vi "test_MSS multiple start stop mismatch1.vi"(8 "Error In":errorcluster) -> (0 "Error Out":errorcluster)   [LabVIEW 2023]
uses:
  Measure and Stimulus Subsystems.lvclass
panel:
  out "Powersensor Chart":waveform(dbl)(graph)
  in  "Stop":bool
  out "Photosensor Chart":waveform(dbl)(graph)
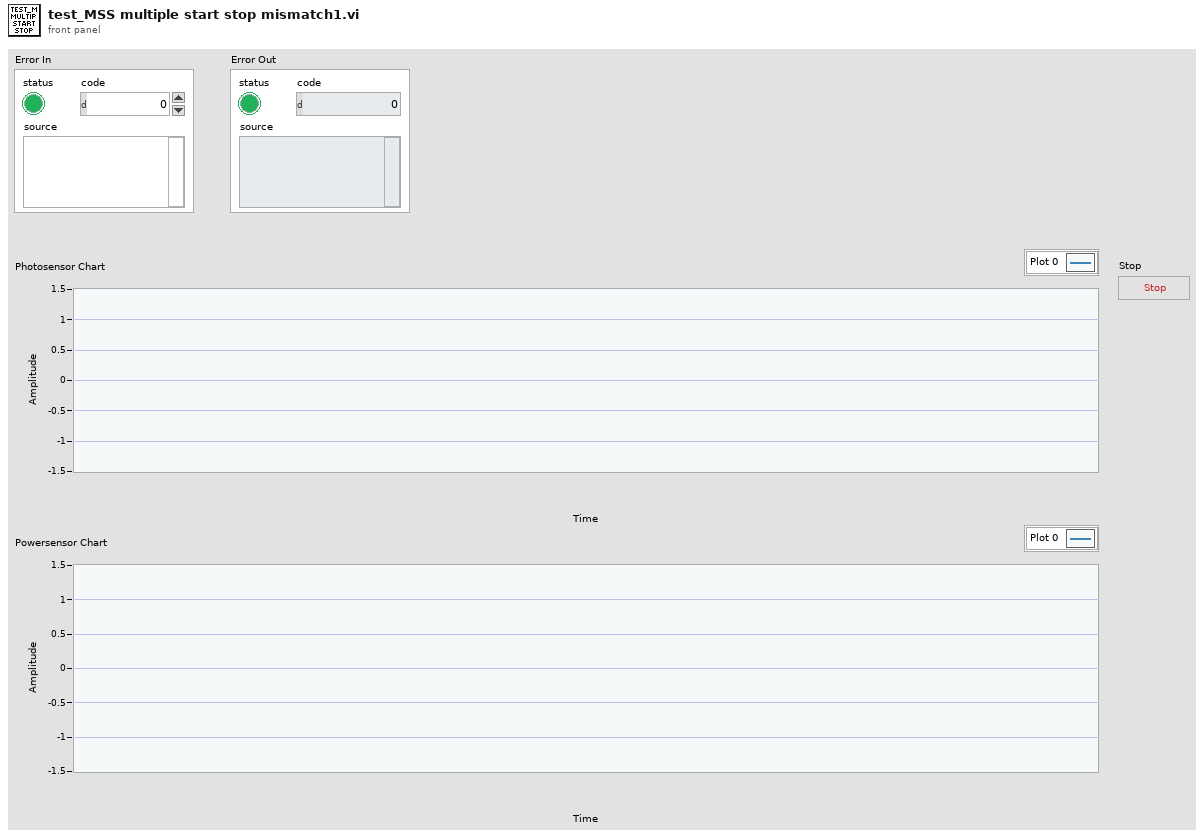
[diagram p1: front panel]
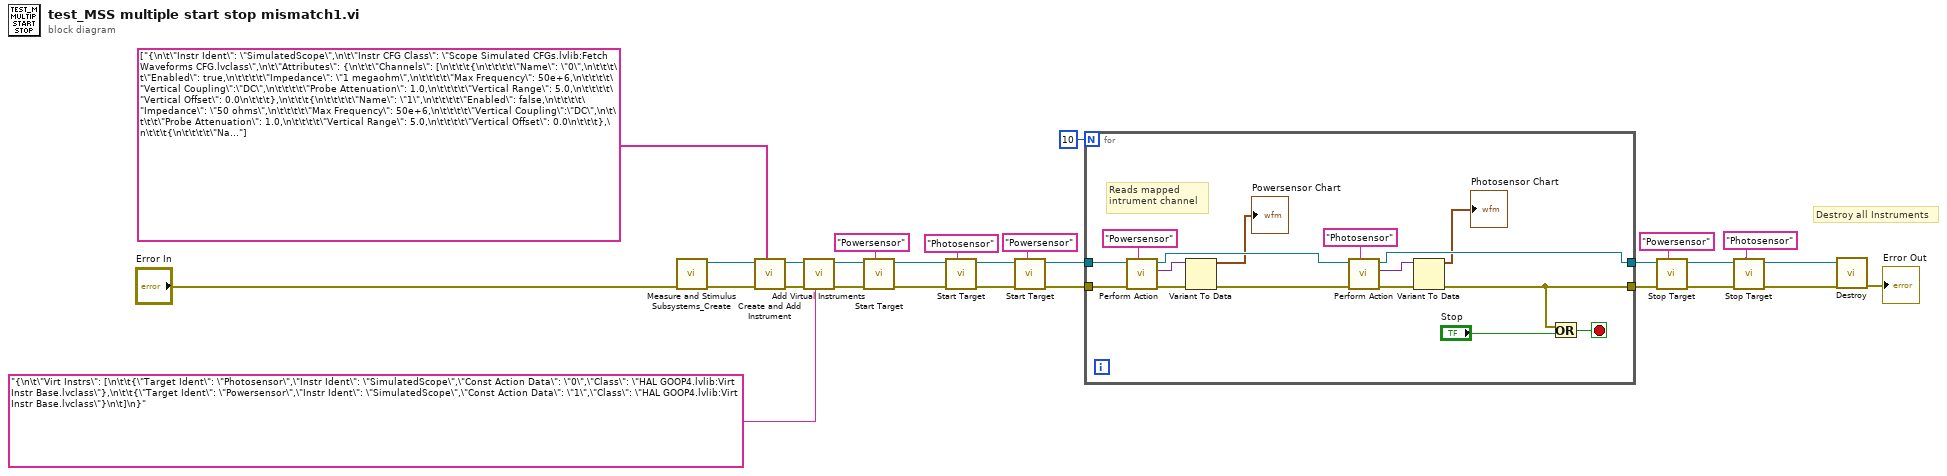
[diagram p0: block diagram]
diagram:
  # "Destroy all Instruments"
  n1 = call "Measure and Stimulus Subsystems_Create.vi"("Error In"="Error In") -> ("Error Out"=w27:errorcluster, "reference out"=w28:refnum<class "Measure and Stimulus Subsystems.lvclass">)  [unwired: 9 in]
  n2 = call "Create and Add Instrument.vi"("Physical Intr Configs"=string[] ["{\n\t\"Instr Ident\": \"SimulatedScope\",\n\t\"Instr CFG Class\": \"Scope Simulated CFGs.lvlib:Fetch Waveforms CFG.lvclass\",\n\t\"Attributes\": {\n\t\t\"Channels\": [\n\t\t\t{\n\t\t\t\t\"Name\": \"0\",\n\t\t\t\t\"Enabled\": true,\n\t\t\t\t\"Impedance\": \"1 megaohm\",\n\t\t\t\t\"Max Frequency\": 50e+6,\n\t\t\t\t\"Vertical Coupling\":\"DC\",\n\t\t\t\t\"Probe Attenuation\": 1.0,\n\t\t\t\t\"Vertical Range\": 5.0,\n\t\t\t\t\"Vertical Offset\": 0.0\n\t\t\t},\n\t\t\t{\n\t\t\t\t\"Name\": \"1\",\n\t\t\t\t\"Enabled\": false,\n\t\t\t\t\"Impedance\": \"50 ohms\",\n\t\t\t\t\"Max Frequency\": 50e+6,\n\t\t\t\t\"Vertical Coupling\":\"DC\",\n\t\t\t\t\"Probe Attenuation\": 1.0,\n\t\t\t\t\"Vertical Range\": 5.0,\n\t\t\t\t\"Vertical Offset\": 0.0\n\t\t\t},\n\t\t\t{\n\t\t\t\t\"Name\": \"2\",\n\t\t\t\t\"Enabled\": false,\n\t\t\t\t\"Impedance\": \"50 ohms\",\n\t\t\t\t\"Max Frequency\": 50e+6,\n\t\t\t\t\"Vertical Coupling\":\"DC\",\n\t\t\t\t\"Probe Attenuation\": 1.0,\n\t\t\t\t\"Vertical Range\": 5.0,\n\t\t\t\t\"Vertical Offset\": 0.0\n\t\t\t},\n\t\t\t{\n\t\t\t\t\"Name\": \"3\",\n\t\t\t\t\"Enabled\": true,\n\t\t\t\t\"Impedance\": \"50 ohms\",\n\t\t\t\t\"Max Frequency\": 50e+6,\n\t\t\t\t\"Vertical Coupling\":\"DC\",\n\t\t\t\t\"Probe Attenuation\": 1.0,\n\t\t\t\t\"Vertical Range\": 1.4,\n\t\t\t\t\"Vertical Offset\": 0.0\n\t\t\t},\n\t\t\t{\n\t\t\t\t\"Name\": \"4\",\n\t\t\t\t\"Enabled\": false,\n\t\t\t\t\"Impedance\": \"50 ohms\",\n\t\t\t\t\"Max Frequency\": 50e+6,\n\t\t\t\t\"Vertical Coupling\":\"DC\",\n\t\t\t\t\"Probe Attenuation\": 1.0,\n\t\t\t\t\"Vertical Range\": 5.0,\n\t\t\t\t\"Vertical Offset\": 0.0\n\t\t\t},\n\t\t\t{\n\t\t\t\t\"Name\": \"5\",\n\t\t\t\t\"Enabled\": false,\n\t\t\t\t\"Impedance\": \"50 ohms\",\n\t\t\t\t\"Max Frequency\": 50e+6,\n\t\t\t\t\"Vertical Coupling\":\"DC\",\n\t\t\t\t\"Probe Attenuation\": 1.0,\n\t\t\t\t\"Vertical Range\": 5.0,\n\t\t\t\t\"Vertical Offset\": 0.0\n\t\t\t},\n\t\t\t{\n\t\t\t\t\"Name\": \"6\",\n\t\t\t\t\"Enabled\": false,\n\t\t\t\t\"Impedance\": \"50 ohms\",\n\t\t\t\t\"Max Frequency\": 50e+6,\n\t\t\t\t\"Vertical Coupling\":\"DC\",\n\t\t\t\t\"Probe Attenuation\": 1.0,\n\t\t\t\t\"Vertical Range\": 5.0,\n\t\t\t\t\"Vertical Offset\": 0.0\n\t\t\t},\n\t\t\t{\n\t\t\t\t\"Name\": \"7\",\n\t\t\t\t\"Enabled\": false,\n\t\t\t\t\"Impedance\": \"50 ohms\",\n\t\t\t\t\"Max Frequency\": 50e+6,\n\t\t\t\t\"Vertical Coupling\":\"DC\",\n\t\t\t\t\"Probe Attenuation\": 1.0,\n\t\t\t\t\"Vertical Range\": 5.0,\n\t\t\t\t\"Vertical Offset\": 0.0\n\t\t\t}\n\t\t],\n\t\t\"Horizontal\": {\n\t\t\t\"Enforce Realtime\": true,\n\t\t\t\"Number of Records\": 1,\n\t\t\t\"Min Sample Rate\": 1e+5,\n\t\t\t\"Reference Position\":50, //percent\n\t\t\t\"Min Record Length\":1e+3\n\t\t},\n\t\t\"Acquire\": {\n\t\t\t\"Type\": \"Normal\",\n\t\t\t\"NumSamples\": 1e+3,\n\t\t\t\"Fetch Relative To\": \"Read Pointer\"\n\t\t},\n\t\t\"Export Signal\": {\n\t\t\t\"Signal Identifier\": \"None\",\n\t\t\t\"Signal\": \"None\",\n\t\t\t\"Output Terminal\": \"None\"\n\t\t},\n\t\t\"Trigger\": {\n\t\t\t\"Type\": \"Immediate\",\n\t\t\t\"Slope\": \"Positive\",\n\t\t\t\"Source\": \"RTSI 0\",\n\t\t\t\"Holdoff\": 0.0,\n\t\t\t\"Delay\": 0.0\n\t\t}\n\t}\n}"], "Error In"=w27, "reference in"=w28) -> ("Error Out"=w23:errorcluster, "reference out"=w9:refnum<class "Measure and Stimulus Subsystems.lvclass">)  [unwired: 7 in]
  n3 = call "Add Virtual Instruments.vi"("<JSON CFG>"="{\n\t\"Virt Instrs\": [\n\t\t{\"Target Ident\": \"Photosensor\",\"Instr Ident\": \"SimulatedScope\",\"Const Action Data\": \"0\",\"Class\": \"HAL GOOP4.lvlib:Virt Instr Base.lvclass\"},\n\t\t{\"Target Ident\": \"Powersensor\",\"Instr Ident\": \"SimulatedScope\",\"Const Action Data\": \"1\",\"Class\": \"HAL GOOP4.lvlib:Virt Instr Base.lvclass\"}\n\t]\n}", "Error In"=w23, "reference in"=w9) -> ("Error Out"=w10:errorcluster, "reference out"=w8:refnum<class "Measure and Stimulus Subsystems.lvclass">)  [unwired: 7 in]
  n4 = call "Start Target.vi"("Target Ident"="Powersensor", "Error In"=w10, "reference in"=w8) -> ("Error Out"=w21:errorcluster, "reference out"=w19:refnum<class "Measure and Stimulus Subsystems.lvclass">)  [unwired: 7 in]
  n5 = call "Start Target.vi"("Target Ident"="Photosensor", "Error In"=w21, "reference in"=w19) -> ("Error Out"=w20:errorcluster, "reference out"=w5:refnum<class "Measure and Stimulus Subsystems.lvclass">)  [unwired: 7 in]
  n6 = call "Start Target.vi"("Target Ident"="Powersensor", "Error In"=w20, "reference in"=w5) -> ("Error Out"=w6:errorcluster, "reference out"=w4:refnum<class "Measure and Stimulus Subsystems.lvclass">)  [unwired: 7 in]
  n7 = for {
    N: 10 -> [_]
    tunnel: w6 -> [w37]
    tunnel: w4 -> [w36]
    tunnel: [w38] -> w15
    tunnel: [w40] -> w25
    stop <- w44 stop-if-true
    # "Reads mapped\nintrument channel"
    n8 = call "Perform Action.vi"("Target Ident"="Powersensor" ("Target Identifier"), "Error In"=w37, "reference in"=w36) -> ("Error Out"=w35:errorcluster, "Output"=w31:variant, "reference out"=w32:refnum<class "Measure and Stimulus Subsystems.lvclass">)  [unwired: 6 in]
    n9 = Variant To Data(error in=w35, Variant=w31) -> (data=→"Powersensor Chart":waveform(dbl), error out=w33:errorcluster)  [unwired: 1 in]
    n10 = call "Perform Action.vi"("Target Ident"="Photosensor" ("Target Identifier"), "Error In"=w33, "reference in"=w32) -> ("Error Out"=w42:errorcluster, "Output"=w39:variant, "reference out"=w38:refnum<class "Measure and Stimulus Subsystems.lvclass">)  [unwired: 6 in]
    n11 = Variant To Data(error in=w42, Variant=w39) -> (data=→"Photosensor Chart":waveform(dbl), error out=w40:errorcluster)  [unwired: 1 in]
    n12 = Or(x=w40, y="Stop") -> (x .or. y?=w44:bool)
  }
  n13 = call "Stop Target.vi"("Target Ident"="Powersensor", "Error In"=w25, "reference in"=w15) -> ("Error Out"=w16:errorcluster, "reference out"=w14:refnum<class "Measure and Stimulus Subsystems.lvclass">)  [unwired: 7 in]
  n14 = call "Stop Target.vi"("Target Ident"="Photosensor", "Error In"=w16, "reference in"=w14) -> ("Error Out"=w1:errorcluster, "reference out"=w2:refnum<class "Measure and Stimulus Subsystems.lvclass">)  [unwired: 7 in]
  n15 = call "Destroy.vi"("Error In"=w1, "reference in"=w2) -> ("Error Out"=→"Error Out":errorcluster)  [unwired: 8 in, 1 out]
